vi "Signal-error.vi"(8 "error in (no error)":errorcluster, 11 "ModComm in":T1) -> (0 "error out":errorcluster, 3 "ModComm out":T1)   [LabVIEW 2013, in "SLMServer.lvlib" / "SLMServer.lvclass"]
uses:
  SLMServer.lvclass
  Object-reference.ctl
  SLMServer.lvclass/SLMServer.ctl
  Read Error log.vi
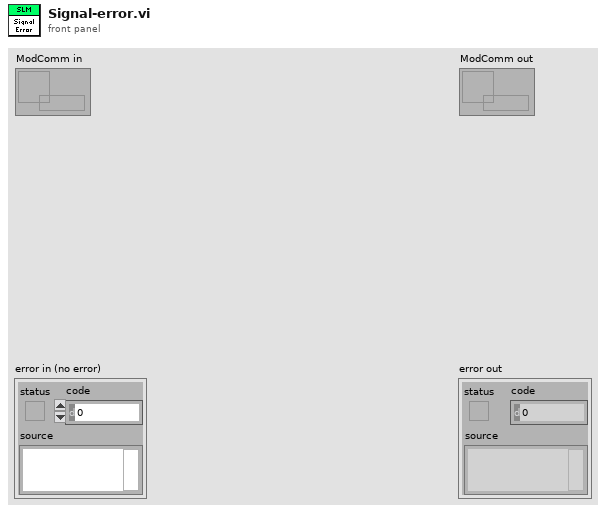
[diagram p1: front panel]
types:
  T1 = typedef "SLMServer.lvlib/SLMServer.lvclass/Object-reference.ctl" = refnum<data-value>
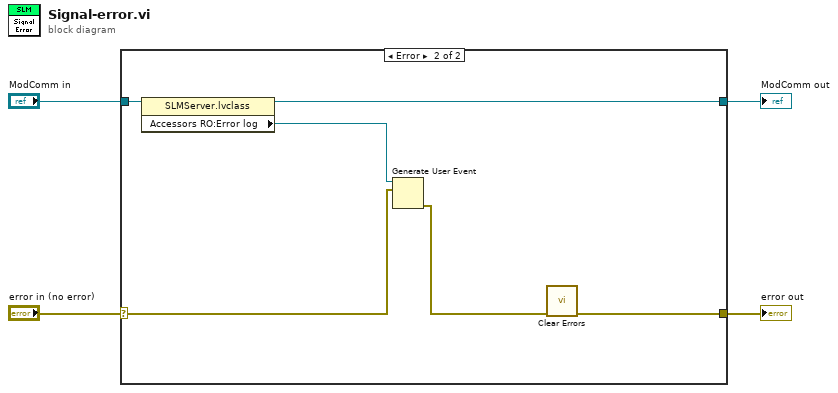
[diagram p0: block diagram]
diagram:
  n1 = case shown="Error" "error in (no error)" {
    selector: "error in (no error)" -> [w6 w9]
    tunnel: "ModComm in" -> [w5 w12]
    tunnel: [w5 w11] -> w3
    tunnel: [w6 w7] -> w2
    frame No Error {
    }
    frame Error {
      n2 = property class="SLMServer.lvclass"(reference=w12) -> (reference out=w11:T1, "Accessors RO:Error log"=w10:refnum<user-event>)  [unwired: 1 in, 1 out]
      n3 = Generate User Event(user event=w10, event data cluster=w9) -> (error out=w8:errorcluster)  [unwired: 2 in, 1 out]
      n4 = call <vilib>:"Clear Errors.vi"("error in (no error)"=w8) -> ("error out"=w7:errorcluster)  [unwired: 6 in]
    }
  }
  "error out" <- w2
  "ModComm out" <- w3
